vi "QueryServer_Start.vi"(7 "error in (no error)":errorcluster, 10 "Server Address":string) -> (0 "error out":errorcluster, 2 "Event Registration Refnum":refnum<event-registration>, 3 "server ref":T2)   [LabVIEW 2019]
uses:
  QueryServer_gRPCid.ctl
  QueryServer_Serverid.ctl
  Debug/labview_query_server.dll
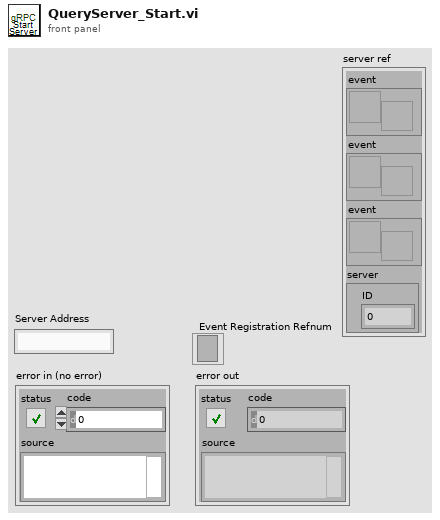
[diagram p1: front panel]
types:
  T1 = typedef "QueryServer_Serverid.ctl" = cluster{"ID":u64}
  T2 = cluster{"event":refnum<user-event>, "event":refnum<user-event>, "event":refnum<user-event>, "server":T1}
  T3 = typedef "QueryServer_gRPCid.ctl" = cluster{"ID":u64}
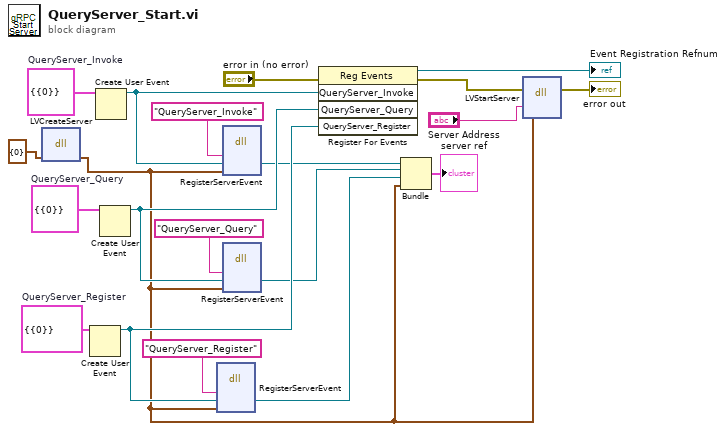
[diagram p0: block diagram]
diagram:
  w13 = cluster{"gRPCid":T3} {"gRPCid"={"ID"=0}}  # QueryServer_Register
  w16 = cluster{"gRPCid":T3} {"gRPCid"={"ID"=0}}  # QueryServer_Query
  w18 = cluster{"gRPCid":T3} {"gRPCid"={"ID"=0}}  # QueryServer_Invoke
  n1 = dll-call lib="C:/dev/labview-grpc-query-server/Debug/labview_query_server.dll" fn="LVCreateServer"("server"=T1 {"ID"=0} ("ServerId")) -> ("server"=w2:T1)  [unwired: 4 in, 2 out]
  n2 = Create User Event(user event datatype=w13) -> (user event=w12:refnum<user-event>)  [unwired: 1 in, 1 out]
  n3 = Create User Event(user event datatype=w18) -> (user event=w20:refnum<user-event>)  [unwired: 1 in, 1 out]
  n4 = Create User Event(user event datatype=w16) -> (user event=w15:refnum<user-event>)  [unwired: 1 in, 1 out]
  n5 = dll-call lib="C:/dev/labview-grpc-query-server/Debug/labview_query_server.dll" fn="RegisterServerEvent"("name"="QueryServer_Register", "event"=w12, "serverid"=w2) -> ("event"=w4:refnum<user-event>)  [unwired: 6 in, 2 out]
  n6 = dll-call lib="C:/dev/labview-grpc-query-server/Debug/labview_query_server.dll" fn="RegisterServerEvent"("name"="QueryServer_Invoke", "event"=w20, "serverid"=w2) -> ("event"=w6:refnum<user-event>)  [unwired: 6 in, 2 out]
  n7 = dll-call lib="C:/dev/labview-grpc-query-server/Debug/labview_query_server.dll" fn="RegisterServerEvent"("name"="QueryServer_Query", "event"=w15, "serverid"=w2) -> ("event"=w5:refnum<user-event>)  [unwired: 6 in, 2 out]
  n8 = register-events(error in="error in (no error)", w20, w15, w12) -> (reference out=→"Event Registration Refnum":refnum<event-registration>, error out=w9:errorcluster)  [unwired: 1 in]
  n9 = Bundle("event"=w6, "event"=w5, "event"=w4, "server"=w2) -> (→"server ref":T2)  [unwired: 1 in]
  n10 = dll-call lib="C:/dev/labview-grpc-query-server/Debug/labview_query_server.dll" fn="LVStartServer"(error in=w9, "serveraddress"="Server Address", "serverid"=w2) -> (error out=→"error out":errorcluster)  [unwired: 5 in, 1 out]
